vi "TcpClient.vi"(7 "DataToSend":string, 9 "OpenTimeout [ms] (5000)":i32=5000, 10 "Port":u16, 11 "Address (127.0.0.1)":string="127.0.0.1") -> (0 "error out":errorcluster, 5 "ReceivedData":string)   [LabVIEW 2021]
uses:
  TcpClient/TcpClient.lvclass
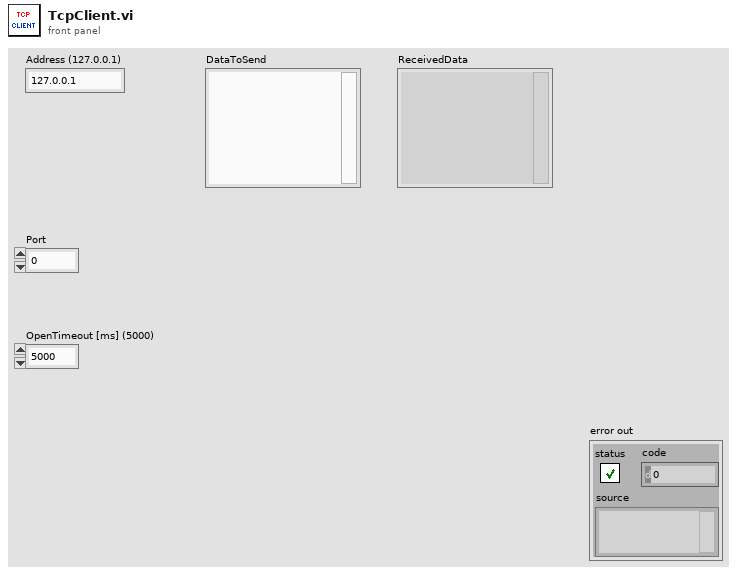
[diagram p1: front panel]
types:
  T1 = enum16{"Standard", "Buffered", "CRLF", "Immediate"}
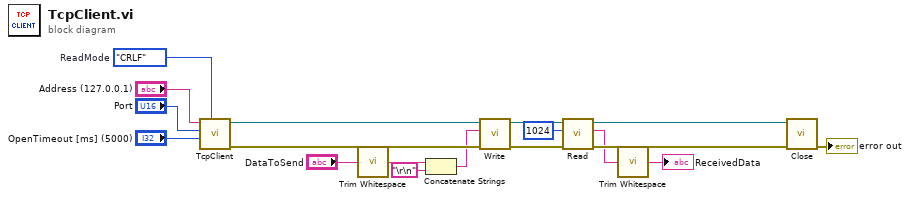
[diagram p0: block diagram]
diagram:
  w6 = T1."CRLF"  # ReadMode
  n1 = call "TcpClient.vi"("ReadMode (Standard)"=w6, "OpenTimeout [ms] (5000)"="OpenTimeout [ms] (5000)", "Port"="Port", "Address (127.0.0.1)"="Address (127.0.0.1)") -> ("error out"=w18:errorcluster, "TcpClient"=w8:refnum<class "TcpClient.lvclass">)  [unwired: 6 in]
  n2 = call <vilib>:"Trim Whitespace.vi"("string"="DataToSend") -> ("trimmed string"=w1:string)  [unwired: 1 in]
  n3 = Concatenate Strings(w1, "\r\n") -> (w4:string)
  n4 = call-dynamic "Write.vi"("error in (no error)"=w18, "Data"=w4, "TcpClient in"=w8) -> ("error out"=w9:errorcluster, "TcpClient out"=w7:refnum<class "TcpClient.lvclass">)  [unwired: 7 in]
  n5 = call-dynamic "Read.vi"("error in (no error)"=w9, "BytesToRead"=1024, "TcpClient in"=w7) -> ("error out"=w17:errorcluster, "Data"=w11:string, "TcpClient out"=w16:refnum<class "TcpClient.lvclass">)  [unwired: 6 in]
  n6 = call <vilib>:"Trim Whitespace.vi"("string"=w11) -> ("trimmed string"=→"ReceivedData":string)  [unwired: 1 in]
  n7 = call-dynamic "Close.vi"("error in (no error)"=w17, "TcpSocket in"=w16) -> ("error out"=→"error out":errorcluster)  [unwired: 8 in, 1 out]
